vi "mes~设备状态采集.vi"(7 "faultCodes":string[](array[string]), 8 "error in":errorcluster caption="错误输入（无错误）", 10 "RecordDate":string, 11 "设备状态":string caption="设备状态:") -> (0 "error out":errorcluster caption="错误输出", 1 "ErrorMessage":string, 2 "设备状态采集成功":bool)   [LabVIEW 2020]
uses:
  ctl/SendEquipStatusCollect.ctl
  ctl/ReceiveEquipStatusCollect.ctl
  Global.vi
panel:
  in  "Headers":string[][](array[string])=[["Content-Type", "text/xml;charset=UTF-8"], ["SOAPAction", "\"http://tempuri.org/ICalbEquipStatusCollectWcf/EquipStatusCollect\""], ["Connection", "Keep-Alive"], ["User-Agent", "Apache-HttpClient/4.1.1 (java 1.5)"]]
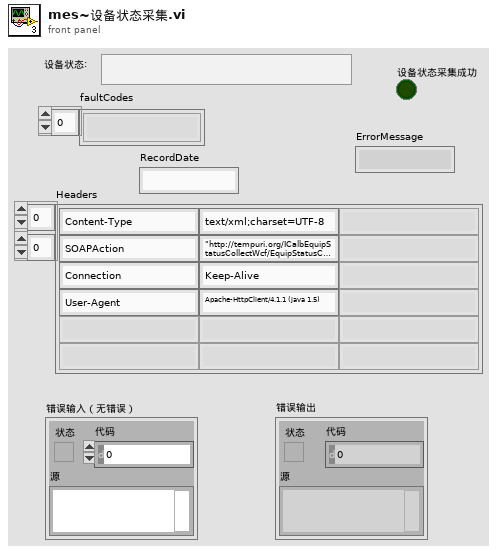
[diagram p1: front panel]
types:
  T1 = typedef "SendEquipStatusCollect.ctl" = cluster{"#attributes":cluster{"xmlns:soapenv":string, "xmlns:tem":string, "xmlns:cal":string, "xmlns:arr":string}, "soapenv:Header":string, "soapenv:Body":cluster{"tem:EquipStatusCollect":cluster{"tem:vo":cluster{"cal:equipNum":string, "cal:faultCodes":cluster{"arr:string":string[]}, "cal:recordDate":string, "cal:remarks":string, "cal:siteCode":string, "cal:statusCode":string, "cal:userName":string}}}}
  T2 = cluster{"接口地址(URL)":string, "用户登录":string, "产品进站":string, "参数采集":string, "产品出站":string, "设备状态":string, "设备编号(equipNum)":string, "站点名称(siteCode)":string, "生产类型(productType)":string, "追溯编号(traceCode)":string}
  T3 = typedef "ReceiveEquipStatusCollect.ctl" = cluster{"#attributes":cluster{"xmlns:s":string}, "s:Body":cluster{"EquipStatusCollectResponse":cluster{"#attributes":cluster{"xmlns":string}, "EquipStatusCollectResult":cluster{"#attributes":cluster{"xmlns:a":string, "xmlns:i":string}, "a:ErrorCode":string, "a:ErrorMessage":string, "a:Success":string}}}}
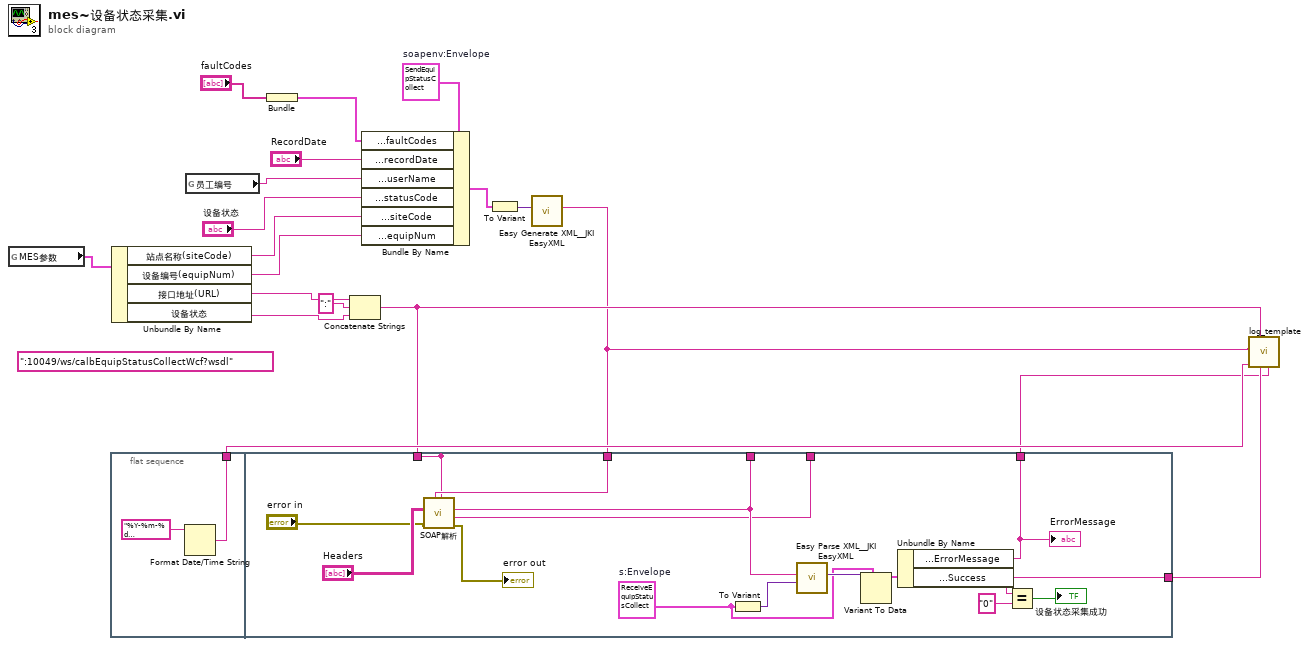
[diagram p0: block diagram]
diagram:
  w11 = T1 {"#attributes"={"xmlns:soapenv"="http://schemas.xmlsoap.org/soap/envelope/", "xmlns:tem"="http://tempuri.org/", "xmlns:cal"="http://schemas.datacontract.org/2004/07/CalbEquipStatusCollectService", "xmlns:arr"="http://schemas.microsoft.com/2003/10/Serialization/Arrays"}, "soapenv:Header"="", "soapenv:Body"={"tem:EquipStatusCollect"={"tem:vo"={"cal:equipNum"="", "cal:faultCodes"={"arr:string"=[]}, "cal:recordDate"="", "cal:remarks"="", "cal:siteCode"="", "cal:statusCode"="", "cal:userName"=""}}}}  # soapenv:Envelope
  (unwired) ":10049/ws/calbEquipStatusCollectWcf?wsdl"
  n1 = global read "Global.vi" "MES参数"() -> (w15:T2)
  n2 = flat-sequence {
    tunnel: [w20] -> w5
    tunnel: w1 -> [w31]
    tunnel: [w30] -> _
    tunnel: [w28] -> _
    tunnel: [w29] -> _
    tunnel: w2 -> [w28]
    tunnel: [w23] -> w3
    tunnel: [w22] -> w4
    frame #0 {
      n3 = Format Date/Time String(time format string (%c)="%Y-%m-%d %H:%M:%S%3u-->" ("EndTime")) -> (date/time string=w20:string)  [unwired: 2 in]
    }
    frame #1 {
      w25 = T3 {"#attributes"={"xmlns:s"="1.0"}, "s:Body"={"EquipStatusCollectResponse"={"#attributes"={"xmlns"=""}, "EquipStatusCollectResult"={"#attributes"={"xmlns:a"="", "xmlns:i"=""}, "a:ErrorCode"="", "a:ErrorMessage"="", "a:Success"=""}}}}  # s:Envelope
      n4 = call "SOAP解析.vi"("DATA"=w31, "错误输入（无错误）"="error in", "Headers"="Headers", "URL"=w28) -> ("错误输出"=→"error out":errorcluster, "headers"=w29:string, "body"=w30:string)  [unwired: 5 in]
      n5 = To Variant(anything=w25) -> (Variant=w36:variant)
      n6 = call <vilib>:"Easy Parse XML__JKI EasyXML.vi"("LabVIEW Data (Type)"=w36, "XML String"=w30) -> ("LabVIEW Data"=w35:variant)  [unwired: 8 in, 1 out]
      n7 = Variant To Data(type=w25, Variant=w35) -> (data=w34:T3)  [unwired: 1 in, 1 out]
      n8 = Unbundle By Name(w34) -> ("s:Body.EquipStatusCollectResponse.EquipStatusCollectResult.a:ErrorMessage"=w23:string, "s:Body.EquipStatusCollectResponse.EquipStatusCollectResult.a:Success"=w22:string)
      "ErrorMessage" <- w23
      n9 = Equal?(x=w22, y="0") -> (x = y?=→"设备状态采集成功":bool)
    }
  }
  n10 = Unbundle By Name(w15) -> ("站点名称(siteCode)"=w16:string, "设备编号(equipNum)"=w17:string, "接口地址(URL)"=w14:string, "设备状态"=w7:string)
  n11 = global read "Global.vi" "员工编号"() -> (w13:string)
  n12 = Bundle("faultCodes"="faultCodes") -> (w10:cluster{"faultCodes":string[]})  [unwired: 1 in]
  n13 = Concatenate Strings(w14, ":" ("字符串"), w7) -> (w2:string)
  n14 = Bundle By Name(cluster=w11, "soapenv:Body.tem:EquipStatusCollect.tem:vo.cal:faultCodes"=w10, "soapenv:Body.tem:EquipStatusCollect.tem:vo.cal:recordDate"="RecordDate", "soapenv:Body.tem:EquipStatusCollect.tem:vo.cal:userName"=w13, "soapenv:Body.tem:EquipStatusCollect.tem:vo.cal:statusCode"="设备状态", "soapenv:Body.tem:EquipStatusCollect.tem:vo.cal:siteCode"=w16, "soapenv:Body.tem:EquipStatusCollect.tem:vo.cal:equipNum"=w17) -> (w19:T1)
  n15 = To Variant(anything=w19) -> (Variant=w18:variant)
  n16 = call <vilib>:"Easy Generate XML__JKI EasyXML.vi"("LabVIEW Data"=w18) -> ("XML String"=w1:string)  [unwired: 9 in, 1 out]
  n17 = call "log_template.vi"("接收报文"=w3, "a:Success"=w4, "URL"=w2, "StartTime"=w5, "发送报文"=w1) -> ()  [unwired: 7 in]
